vi "模拟器自动控制程序.vi"() -> ()   [LabVIEW 2012]
uses:
  <vilib>/Utility/error.llb/DialogType.ctl
  <vilib>/Platform/TimedLoop/XDataNode/timing_clust.ctl
  <vilib>/Platform/TimedLoop/XDataNode/nitl_modes.ctl
  <vilib>/Platform/TimedLoop/XDataNode/wakeup.ctl
  <vilib>/Instr/_visa.llb/VISA Configure Serial Port (Instr).vi
  <vilib>/DAQmx/create/channels.llb/DAQmx Create Channel (DO-Digital Output).vi
  <vilib>/Analysis/Matrix/Numeric/Conversions/Array To Matrix - RA2.vi
  <vilib>/Utility/file.llb/Write To Spreadsheet File (DBL).vi
  <vilib>/Platform/TimedLoop/XDataNode/XDataNode.xnode
  <vilib>/Platform/TimedLoop/XDataNode/XDNodeRunTimeDep.lvlib
  <vilib>/Analysis/Matrix/NI_Matrix.lvlib
  <vilib>/vision/NI_Vision_Development_Module.lvlib
  <vilib>/Analysis/NI_AALBase.lvlib
panel:
  out "Truster4":bool
  out "Truster 8":bool
  out "Truster  3":bool
  out "Truster 7":bool
  out "Truster 5":bool
  out "Truster  2":bool
  out "Truster 6":bool
  out "Truster1":bool
  out "alpha (deg)":dbl
  out "定位点信息":T1(array[cluster]) {"Aspect Ratio" format="%.2f"; "Orientation" format="%.2f"; "Area" format="%.2f"; "Object Center"."Y" format="%.2f"; "Object Center"."X" format="%.2f"}
  out "alpha":dbl
  out "计时参数":dbl
  in  "卫星模拟器":enum32{"初始化", "运行监测"}(tab)
  out "读取缓冲区":string
  out "电流校正模式":bool
  out "软件使能":bool caption="软件使能(启动/停止)"
  out "电流校正中":bool caption="电流校正完成"
  out "E2PROM初始化结果":bool
  out "E2初始化完成":bool
  out "串口通信错误":bool caption="串口通信故障"
  out "发送指令":string
  out "控制命令":string
  out "电机已启动":bool
  in  "采样率":i64=10
  in  "限制转速":dbl=500.0
  in  "ID号":u8=255 step=1 format="%#.0f"
  in  "最高转速":dbl=500.0
  in  "PWM周期":dbl=1599.0
  in  "最大力矩":dbl=2047.0
  in  "stop bits (10: 1 bit)":u16(ring)=10 caption="停止位" items=["1.0"=10, "1.5"=15, "2.0"=20]
  out "串口状态":bool
  in  "端口选择":refnum<visa-resource-name>="COM1"
  in  "波特率":u16(ring)=10 items=["   300", "   600", "   1200", "   2400", "   4800   ", "   9600", "   19200", "   38400", "   43000", "   56000", "   57600", "   115200"]
  in  "校验":enum16{"None", "Odd", "Even"}(ring)=enum."Even"
  in  "数据位":u16=8
  in  "打开":bool caption="stop"
  out "轨控信号":dbl
  in  "姿轨控开始":bool
  out "转速模式":bool
  out "转矩模式":bool
  out "故障":bool
  out "启停状态":bool
  in  "所需转角":dbl
  in  "存储波形":bool
  in  "显示波形 停止显示":bool
  in  "开始记录":bool
  out "动量轮转矩":dbl format="%#_6f"
  out "动量轮转速":dbl format="%#_4f"
  out "X速率(cm/s)":dbl
  out "Y速率(cm/s)":dbl
  out "Y偏移量 (cm)":dbl
  out "X偏移量 (cm)":dbl
  out "相对偏角(deg)":dbl
  out "角速度(deg/s)":dbl
  out "设备ID":u8=255
  in  "模式选择":u16(ring)=1 items=["电流校正模式", "转矩模式", "转速模式", "开环测试模式"]
  in  "模式选择":bool
  in  "写指令字":dbl
  in  "停止电机":bool
  in  "启动电机":bool
  out "波形图":cluster{"转矩反馈":dbl, "转速反馈":dbl}(graph)
  in  "所需X":dbl
  in  "退出程序":bool caption="停止电机 2"
  in  "Floating":bool
  in  "缩放比例 (像素/cm)":dbl=4.099468
  in  "X中心校正":dbl
  in  "Y中心校正":dbl
  in  "所需Y":dbl
  out "x >= y?":bool
  out "数值":dbl
  out "输出数组 6":dbl[](array[numeric])
  out "输出数组 7":dbl[](array[numeric])
  out "输出数组 10":dbl[](array[numeric])
  out "无符号字节数组 2":u8[](array[numeric])
  # "状态"
  # "设置"
  # "控制信号"
  # "参数确定"
  # "状态显示"
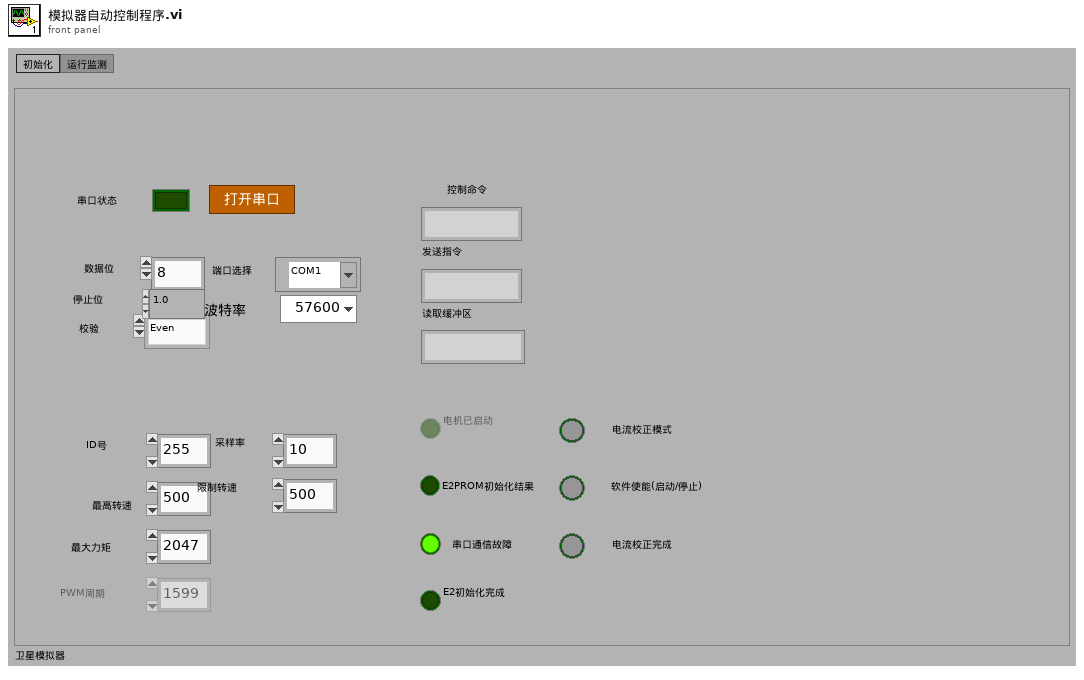
[diagram p1: front panel]
types:
  T1 = cluster{"Object Center":cluster{"X":sgl, "Y":sgl}, "Bounding Box":cluster{"X Left":i32, "Y Top":i32, "X Right":i32, "Y Bottom":i32}, "Area":sgl, "Orientation":sgl, "Aspect Ratio":sgl, "Nb Holes":i32}[]
  T2 = typedef "XDNodeRunTimeDep.lvlib/timing_clust.ctl" = cluster{"Expected End [f-1]":u64, "Actual End [f-1]":u64, "Finished Late? [f-1]":bool, "Expected End [i-1]":u64, "Actual End [i-1]":u64, "Finished Late? [i-1]":bool, "Expected Start [i]":u64, "Actual Start [i]":u64, "Expected Start [f]":u64, "Actual Start [f]":u64, "Source Name":string, "Structure Name":string, "Period":i64, "Deadline":i64, "Offset":i64, "Start":i64, "Priority":i32, "Timeout":i32, "Mode":T3, "Wakeup Reason":T4, "Error":errorcluster, "Source Type":string, "Secondary Source Type":string, "Global End Time":u64, "Global Start Time":u64, "Frame Duration":u64, "Iteration Duration":u64, "Assigned CPU":i32, "I/O Scan Engine Mode":u32}
  T3 = typedef "XDNodeRunTimeDep.lvlib/nitl_modes.ctl" = enum32{"No Change", "Process missed periods, maintain original phase", "Discard missed periods, maintain original phase", "Process missed periods, ignore original phase", "Discard missed periods, ignore original phase"}
  T4 = typedef "XDNodeRunTimeDep.lvlib/wakeup.ctl" = enum32{"Normal", "Aborted", "Asynchronous wakeup", "Timing source error", "Timed loop error", "Timeout"}
  T5 = cluster{"Objects":u16, "Threshold":i32, "Reject Border":bool, "Fill Holes":bool, "Min Object Size":bool, "Min Size":i32, "Max Object Size":bool, "Max Size":i32, "Show Search Area":bool, "Show Center":bool, "Show Bounding Box":bool}
  T6 = typedef "DialogType.ctl" = u16
  T7 = typedef "NI_Matrix.lvlib/RealMatrix.ctl" = dbl[][]
  T8 = typedef "IMAQ Image.ctl" = refnum<image>
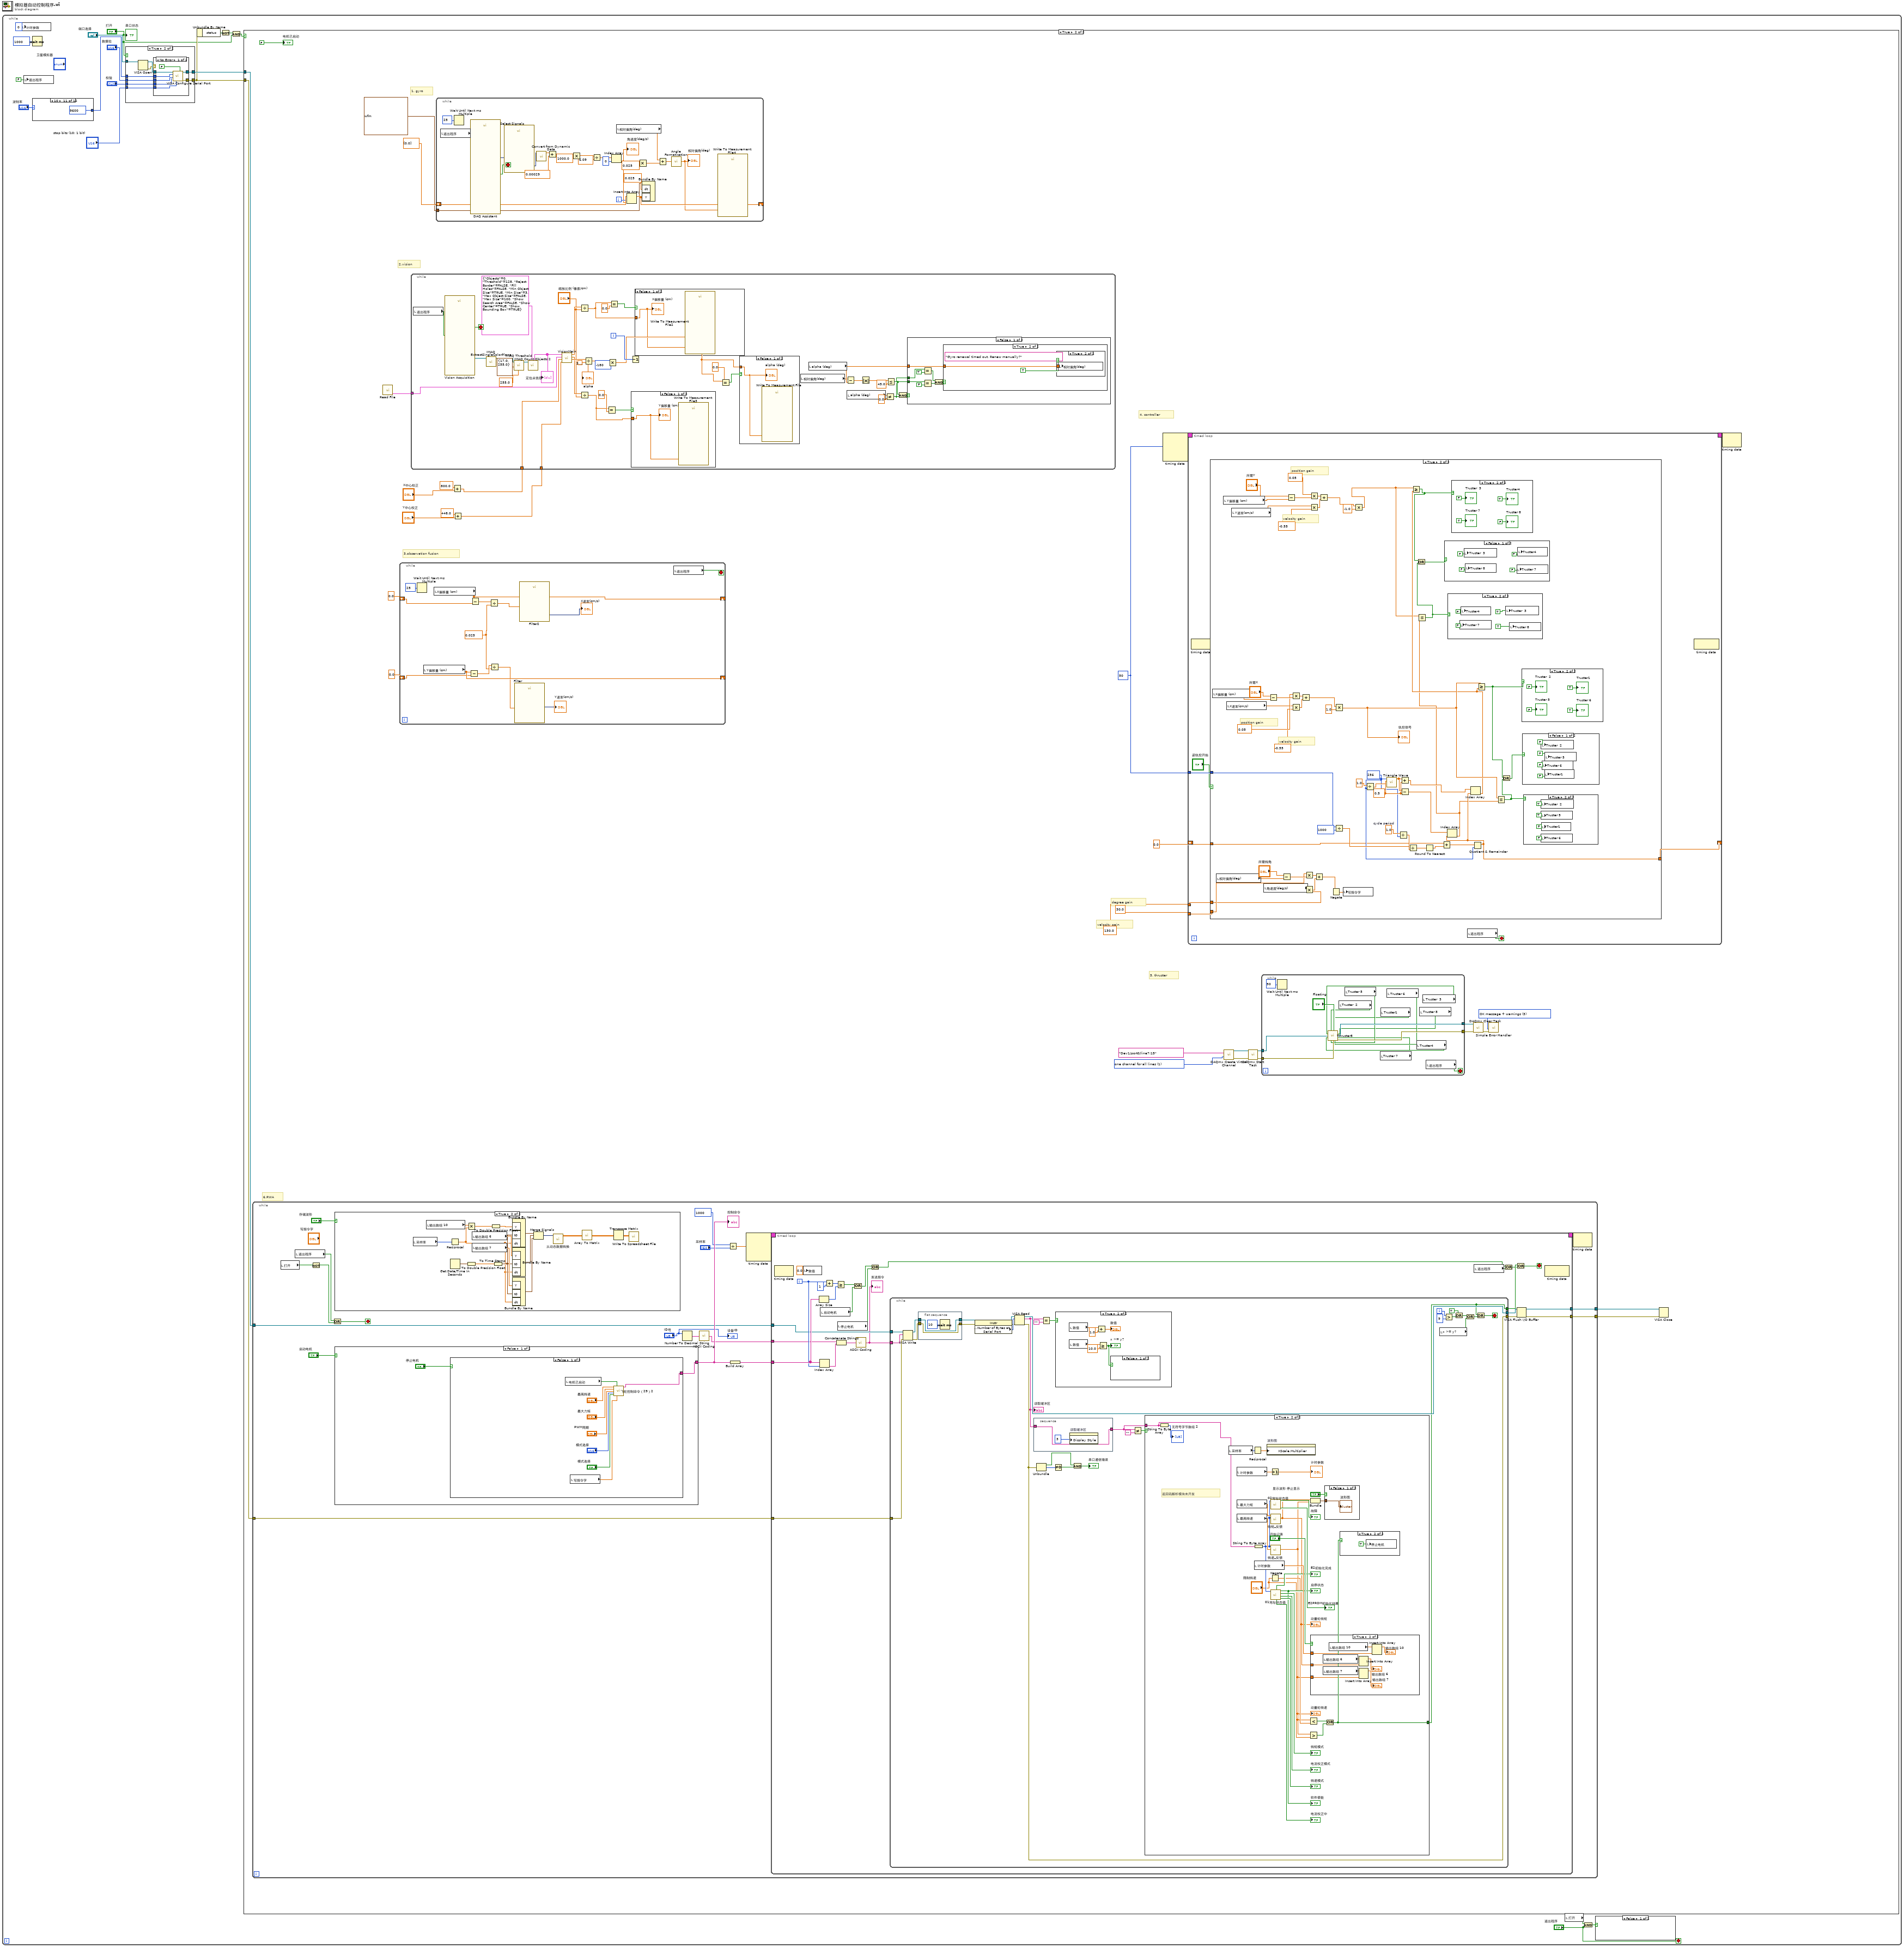
[diagram p0: block diagram]
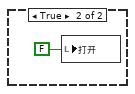
[diagram p2: hidden frame]
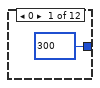
[diagram p5: hidden frame]
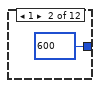
[diagram p6: hidden frame]
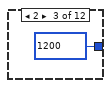
[diagram p7: hidden frame]
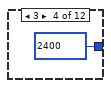
[diagram p8: hidden frame]
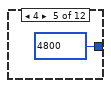
[diagram p9: hidden frame]
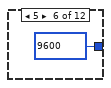
[diagram p10: hidden frame]
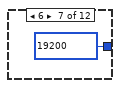
[diagram p11: hidden frame]
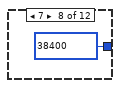
[diagram p12: hidden frame]
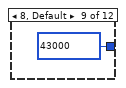
[diagram p13: hidden frame]
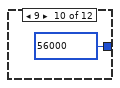
[diagram p14: hidden frame]
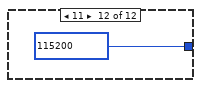
[diagram p15: hidden frame]
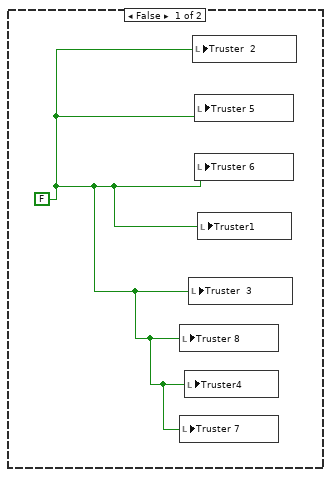
[diagram p17: hidden frame]
diagram:
  n1 = while {
    stop <- "退出程序" stop-if-true
    n2 = local write "计时参数"(0) -> ()
    n3 = local write "退出程序"(FALSE ("退出程序")) -> ()
    n4 = Wait (ms)(milliseconds to wait=u32 1000 ("等待时间（毫秒）")) -> ()  [unwired: 1 out]
    n5 = case shown="10" "波特率" {
      tunnel: [300 600 1200 2400 4800 9600 19200 38400 43000 56000 9600 115200] -> w17
      frame 0 {
      }
      frame 1 {
      }
      frame 2 {
      }
      frame 3 {
      }
      frame 4 {
      }
      frame 5 {
      }
      frame 6 {
      }
      frame 7 {
      }
      frame 8, Default {
      }
      frame 9 {
      }
      frame 10 {
      }
      frame 11 {
      }
    }
    n6 = case shown="True" "打开" {
      tunnel: w17 -> [_ w28]
      tunnel: "数据位" -> [_ w27]
      tunnel: "校验" -> [_ w26]
      tunnel: "端口选择" -> [_ w25]
      tunnel: [_ w22] -> w7
      tunnel: [_ w21] -> w6
      tunnel: "stop bits (10: 1 bit)" -> [_ w20]
      frame False {
      }
      frame True {
        n7 = VISA Open(VISA resource name=w25) -> (VISA resource name=w24:refnum<visa-resource-name>, error out=w23:errorcluster)  [unwired: 1 in, 3 out]
        n8 = case shown="No Error" w23 {
          tunnel: w28 -> [w36 _]
          tunnel: w27 -> [w35 _]
          tunnel: w26 -> [w34 _]
          tunnel: w24 -> [w33 _]
          tunnel: [w32 _] -> w22
          tunnel: [w31 _] -> w21
          tunnel: w20 -> [w30 _]
          frame No Error {
            n9 = call-poly "VISA Configure Serial Port"("VISA resource name"=w33, "Enable Termination\nChar (T)"=FALSE ("Enable Termination\nChar (T)"), "baud rate (9600)"=w36, "data bits (8)"=w35, "parity (0:none)"=w34, "stop bits (10: 1 bit)"=w30) -> ("VISA resource name out"=w32:refnum<visa-resource-name>, "error out"=w31:errorcluster)  [unwired: 2 in, 6 out]
          }
          frame Error {
          }
        }
      }
    }
    n10 = Unbundle By Name(w6) -> ("status"=w12:bool)
    n11 = Not(x=w12) -> (.not. x?=w11:bool)
    n12 = And(x=w11, y="打开") -> (x .and. y?=w8:bool)
    n13 = case shown="True" w8 {
      tunnel: w7 -> [_ w77]
      tunnel: w6 -> [_ w76]
      frame False {
      }
      frame True {
        w55 = 1 items=["one channel for each line", "one channel for all lines"] ("line grouping")
        w57 = T6 3 items=["no dialog", "OK message", "continue or stop message", "OK message + warnings", "continue/stop + warnings"] ("type of dialog (OK msg:1)")
        w51 = 50
        # "5. thruster"
        # "6.RWA"
        # "4. controller"
        # "3.observation fusion"
        # "2.vision"
        # "1. gyro"
        # "velocity gain"
        # "degree gain"
        n14 = while {
          tunnel: [w292] -> w79
          tunnel: [w291] -> w78
          tunnel: w77 -> [w290]
          tunnel: w76 -> [w289]
          stop <- w285 stop-if-true
          n15 = local read "打开"() -> (w288:bool)
          n16 = local read "退出程序"() -> (w287:bool)
          n17 = Not(x=w288) -> (.not. x?=w286:bool)
          n18 = Or(x=w287, y=w286) -> (x .or. y?=w285:bool)
          n19 = case shown="True" "存储波形" {
            frame False {
            }
            frame True {
              n20 = local read "采样率"() -> (w314:i64)
              n21 = local read "输出数组 10"() -> (w307:dbl[])
              n22 = Reciprocal(x=w314) -> (1/x=w309:dbl)
              n23 = Get Date/Time In Seconds() -> (seconds since 1Jan1904=w318:timestamp)
              n24 = Multiply(x=w307, y=w309) -> (x*y=w308:dbl[])
              n25 = To Double Precision Float(number=w318) -> (double precision float=w317:dbl)
              n26 = local read "输出数组 6"() -> (w316:dbl[])
              n27 = local read "输出数组 7"() -> (w315:dbl[])
              n28 = To Double Precision Float(number=w308) -> (double precision float=w306:dbl[])
              n29 = To Time Stamp(1:w317) -> (0:w310:timestamp)
              n30 = Bundle By Name("Y"=w306, "t0"=w310, "dt"=w309) -> (w311:waveform(dbl))  [unwired: 1 out]
              n31 = Bundle By Name("Y"=w316, "t0"=w310, "dt"=w309) -> (w312:waveform(dbl))  [unwired: 1 out]
              n32 = Bundle By Name("Y"=w315, "t0"=w310, "dt"=w309) -> (w313:waveform(dbl))  [unwired: 1 out]
              n33 = Merge Signals(w311, w312, w313) -> (w305:dynamicdata)
              n34 = call "从动态数据转换"("Dynamic Data Type"=w305) -> ("Array"=w304:dbl[][])  [unwired: 3 in]
              n35 = call-poly <vilib>:"Array To Matrix.vi"("Real 2D Array"=w304) -> ("Real Matrix"=w303:T7)
              n36 = Transpose Matrix(1:w303) -> (0:w302:T7)
              n37 = call-poly <vilib>:"Write To Spreadsheet File.vi"("2D data"=w302) -> ()  [unwired: 7 in, 1 out]
            }
          }
          n38 = case shown="False" "启动电机" {
            tunnel: [w434 w449] -> w300
            frame False {
              n39 = case shown="False" "停止电机" {
                tunnel: [w442 "v0"] -> w434
                frame False {
                  n40 = local read "电机已启动"() -> (w436:bool)
                  n41 = local read "写指令字"() -> (w435:dbl)
                  n42 = call "飞轮控制命令（29）2.vi"("最高转速"="最高转速", "电机启动控制指令"=w436, "力矩最大值(uNm)"="最大力矩", "pwmperiod"="PWM周期", "模式选择"="模式选择", "模式确定"="模式选择", "写指令字"=w435) -> ("字符串"=w442:string)  [unwired: 8 in]
                }
                frame True {
                  n43 = local write "电机已启动"(FALSE) -> ()
                  n44 = local write "启动电机"(FALSE ("停止电机")) -> ()
                  n45 = local write "停止电机"(FALSE ("停止电机")) -> ()
                }
              }
            }
            frame True {
              n46 = local write "电机已启动"(TRUE) -> ()
              n47 = local write "启动电机"(FALSE) -> ()
              n48 = call <vilib>:"Space Constant.vi"() -> ("String"=w453:string)
              n49 = Concatenate Strings(w453, "05" ("字符串"), w453, "22" ("字符串"), w453, "01" ("字符串")) -> (w449:string)
            }
          }
          "控制命令" <- w300
          n50 = Number To Decimal String(number="ID号") -> (decimal integer string=w284:string)  [unwired: 1 in]
          n51 = call "ASCII Coding.vi"("cmd"=w284) -> ("cmd sent"=w282:string)
          n52 = Divide(x=i64 1000 ("Period"), y="采样率") -> (x/y=w296:dbl)
          n53 = Build Array(w300) -> (w297:string[])
          n54 = node-c288(w296) -> (w299:T2)  [unwired: 3 in]
          n55 = timed-loop {
            timing: w299 -> [_]
            timing-out: [_] -> w298
            tunnel: w297 -> [w340]
            tunnel: w282 -> [w336]
            tunnel: [w333] -> w292
            tunnel: [w332] -> w291
            tunnel: w290 -> [w331]
            tunnel: w289 -> [w330]
            i -> [w339]
            stop <- w321 stop-if-true
            n56 = node-c288() -> ()  [unwired: 1 in, 1 out]
            n57 = local write "数值"(0.0 ("y")) -> ()
            n58 = Array Size(array=w340) -> (size(s)=w342:i32)
            n59 = Index Array(array=w340, index=w339) -> (element=w341:string)
            n60 = local read "启动电机"() -> (w328:bool)
            n61 = Add(x=w339, y=1) -> (x+y=w343:i32)
            n62 = Greater Or Equal?(x=w343, y=w342) -> (x >= y?=w329:bool)
            n63 = Concatenate Strings(w336, w341) -> (w320:string)
            n64 = local read "停止电机"() -> (w327:bool)
            n65 = Or(x=w329, y=w328) -> (x .or. y?=w326:bool)
            n66 = call "ASCII Coding.vi"("cmd"=w320) -> ("cmd sent"=w319:string)
            "发送指令" <- w319
            n67 = Or(x=w326, y=w327) -> (x .or. y?=w324:bool)
            n68 = while {
              tunnel: [w371] -> w334
              tunnel: [w361] -> w335
              tunnel: w319 -> [w365]
              tunnel: w331 -> [w347]
              tunnel: w330 -> [w346]
              tunnel: [w345] -> w323
              i -> [w370]
              stop <- w354 stop-if-true
              n69 = VISA Write(VISA resource name=w347, write buffer=w365, error in (no error)=w346) -> (VISA resource name out=w352:refnum<visa-resource-name>, error out=w349:errorcluster)  [unwired: 1 out]
              n70 = flat-sequence {
                tunnel: w352 -> [w377]
                tunnel: [w377] -> w351
                tunnel: [w376] -> w350
                tunnel: w349 -> [w376]
                frame #0 {
                  n71 = Wait (ms)(milliseconds to wait=i64 10 ("Period")) -> ()  [unwired: 1 out]
                }
              }
              n72 = property class="Instr"(reference=w351, error in=w350) -> (reference out=w373:refnum<visa-resource-name>, error out=w372:errorcluster, "Serial Settings:Number of Bytes at Serial Port"=w374:u32)
              n73 = VISA Read(VISA resource name=w373, byte count=w374, error in (no error)=w372) -> (VISA resource name out=w371:refnum<visa-resource-name>, read buffer=w364:string, error out=w361:errorcluster)  [unwired: 1 out]
              "读取缓冲区" <- w364
              n74 = stacked-sequence {
                tunnel: [w418] -> w363
                tunnel: w364 -> [w418]
                frame #0 {
                  n75 = property on="读取缓冲区" class="Str"("Display Style"=u32 3 ("显示样式")) -> ()  [unwired: 2 in, 2 out]
                }
              }
              n76 = Unbundle(w361) -> ("status"=w358:bool, "code"=w360:i32)  [unwired: 1 out]
              n77 = Equal?(x=w364, y="") -> (x = y?=w367:bool)
              n78 = Not Equal To 0?(x=w360) -> (x != 0?=w359:bool)
              n79 = case shown="True" w367 {
                frame False {
                  n80 = local write "数值"(0.0 ("数值")) -> ()
                }
                frame True {
                  n81 = local read "数值"() -> (w420:dbl)
                  n82 = local read "数值"() -> (w425:dbl)
                  n83 = Add(x=w420, y=1.0) -> (x+y=→"数值":dbl)
                  n84 = Greater Or Equal?(x=w425, y=10.0) -> (x >= y?=w423:bool)
                  "x >= y?" <- w423
                  n85 = case shown="False" w423 {
                    frame False {
                    }
                    frame True {
                      n86 = local write "打开"(FALSE) -> ()
                    }
                  }
                }
              }
              n87 = And(x=w358, y=w359) -> (x .and. y?=→"串口通信错误":bool)
              n88 = Not Equal?(x=w363, y="") -> (x != y?=w353:bool)
              n89 = case shown="True" w353 {
                tunnel: w363 -> [_ w405]
                tunnel: [_ w404] -> w345
                frame False {
                }
                frame True {
                  # "返回码解析模块未开发"
                  n90 = String To Byte Array(string=w405) -> (unsigned byte array=→"无符号字节数组 2":u8[])
                  n91 = local read "采样率"() -> (w401:i64)
                  n92 = local read "计时参数"() -> (w398:dbl)
                  n93 = local read "最大力矩"() -> (w386:dbl)
                  n94 = local read "最高转速"() -> (w384:dbl)
                  n95 = Reciprocal(x=w401) -> (1/x=w400:dbl)
                  n96 = String To Byte Array(string=w405) -> (unsigned byte array=w383:u8[])
                  n97 = local read "计时参数"() -> (w395:dbl)
                  n98 = property on="波形图" class="WFChart (strict)"("XScale.Multiplier"=w400) -> ()  [unwired: 2 in, 2 out]
                  n99 = Increment(x=w398) -> (x+1=→"计时参数":dbl)
                  n100 = Negate(x="限制转速") -> (-x=w382:dbl)
                  n101 = call "02地址状态值.vi"("unsigned byte array"=w383) -> ("E2初始化失败"=→"E2PROM初始化结果":bool, "故障"=→"故障":bool)  [unwired: 9 in]
                  n102 = call "转矩_反馈.vi"("unsigned byte array"=w383, "最大转矩"=w386) -> ("转矩反馈"=w385:dbl)  [unwired: 9 in]
                  "动量轮转矩" <- w385
                  n103 = call "转速_反馈.vi"("最高转速"=w384, "unsigned byte array"=w383) -> ("转速反馈"=w381:dbl)  [unwired: 9 in]
                  "动量轮转速" <- w381
                  n104 = call "01地址状态值.vi"("unsigned byte array"=w383) -> ("E2初始化完成"=→"E2初始化完成":bool, "电流校正完成"=→"电流校正中":bool, "启停状态"=→"软件使能" →"启停状态":bool, "转矩模式"=→"转矩模式":bool, "电流校正"=→"电流校正模式":bool, "转速模式"=→"转速模式":bool)  [unwired: 4 in]
                  n105 = Less?(x=w381, y=w382) -> (x < y?=w378:bool)
                  n106 = Greater?(x=w381, y="限制转速") -> (0:w379:bool)
                  n107 = Bundle("转矩反馈"=w385, "转速反馈"=w381) -> (w402:cluster{"转矩反馈":dbl, "转速反馈":dbl})  [unwired: 1 out]
                  n108 = case shown="True" "开始记录" {
                    tunnel: w385 -> [_ w409]
                    tunnel: w381 -> [_ w408]
                    tunnel: w395 -> [_ w407]
                    frame False {
                    }
                    frame True {
                      n109 = local read "输出数组 6"() -> (w414:dbl[])
                      n110 = local read "输出数组 7"() -> (w412:dbl[])
                      n111 = local read "输出数组 10"() -> (w410:dbl[])
                      n112 = Insert Into Array(array=w414, new element=w409) -> (→"输出数组 6":dbl[])  [unwired: 1 in]
                      n113 = Insert Into Array(array=w412, new element=w408) -> (→"输出数组 7":dbl[])  [unwired: 1 in]
                      n114 = Insert Into Array(array=w410, new element=w407) -> (→"输出数组 10":dbl[])  [unwired: 1 in]
                    }
                  }
                  n115 = case shown="False" "显示波形 停止显示" {
                    tunnel: w402 -> [w416 _]
                    frame False {
                      "波形图" <- w416
                    }
                    frame True {
                    }
                  }
                  n116 = Or(x=w378, y=w379) -> (x .or. y?=w404:bool)
                  n117 = case shown="True" w404 {
                    frame False {
                    }
                    frame True {
                      n118 = local write "停止电机"(TRUE ("停止电机")) -> ()
                    }
                  }
                }
              }
              n119 = local read "x >= y?"() -> (w356:bool)
              n120 = Greater?(x=w370, y=9) -> (0:w348:bool)
              n121 = Or(x=TRUE, y=w348) -> (x .or. y?=w366:bool)
              n122 = Or(x=w366, y=w356) -> (x .or. y?=w355:bool)
              n123 = Or(x=w345, y=w355) -> (x .or. y?=w354:bool)
            }
            n124 = local read "退出程序"() -> (w325:bool)
            n125 = Or(x=w324, y=w325) -> (x .or. y?=w322:bool)
            n126 = Or(x=w323, y=w322) -> (x .or. y?=w321:bool)
            n127 = VISA Flush I/O Buffer(VISA resource name=w334, error in (no error)=w335) -> (VISA resource name out=w333:refnum<visa-resource-name>, error out=w332:errorcluster)  [unwired: 1 out]
            n128 = node-c288() -> ()  [unwired: 1 in, 1 out]
          }
          n129 = node-c288(w298) -> ()  [unwired: 1 out]
          "设备ID" <- "ID号"
        }
        n130 = call "Read File.vi"() -> ("Objects"=w74:T1)  [unwired: 1 in, 1 out]
        n131 = while {
          shift-right: [w275] -> _
          shift-left: 0.0 ("X偏移量 (cm)") -> [w274]
          shift-right: [w272] -> _
          shift-left: 0.0 ("Y偏移量 (cm)") -> [w271]
          stop <- w280 stop-if-true
          w273 = 0.025 ("y")
          n132 = Wait Until Next ms Multiple(millisecond multiple=u32 25) -> ()  [unwired: 1 out]
          n133 = local read "Y偏移量 (cm)"() -> (w272:dbl)
          n134 = local read "X偏移量 (cm)"() -> (w275:dbl)
          n135 = Subtract(x=w272, y=w271) -> (x-y=w277:dbl)
          n136 = Subtract(x=w275, y=w274) -> (x-y=w278:dbl)
          n137 = Divide(x=w278, y=w273) -> (x/y=w269:dbl)
          n138 = Divide(x=w277, y=w273) -> (x/y=w270:dbl)
          n139 = call "Filter"("Signal"=w270) -> ("Filtered Signal"=→"Y速率(cm/s)":dynamicdata)  [unwired: 9 in, 1 out]
          n140 = call "Filter2"("Signal"=w269) -> ("Filtered Signal"=→"X速率(cm/s)":dynamicdata)  [unwired: 9 in, 1 out]
          n141 = local read "退出程序"() -> (w280:bool)
        }
        n142 = while {
          shift-right: [w253] -> _
          shift-left: dbl[] [0.0] -> [w254]
          tunnel: waveform(dbl) {"t0"=timestamp(0 s since 1904-01-01), "dt"=1.0, "Y"=[]} ("waveform") -> [w251]
          i -> [w252]
          stop <- w268 stop-if-true
          n143 = local read "退出程序"() -> (w248:bool)
          n144 = Wait Until Next ms Multiple(millisecond multiple=u32 25 ("y")) -> ()  [unwired: 1 out]
          n145 = call "DAQ Assistant"("stop (F)"=w248) -> ("data"=w246:dynamicdata, "stopped"=w268:bool)  [unwired: 15 in, 2 out]
          n146 = call "Select Signals"("Signals"=w246) -> ("Signal Out"=w247:dynamicdata)  [unwired: 9 in, 1 out]
          n147 = call "Convert from Dynamic Data"("Dynamic Data Type"=w247) -> ("Array"=w259:dbl[])  [unwired: 3 in]
          n148 = Add(x=w259, y=0.00029) -> (x+y=w257:dbl[])
          n149 = Multiply(x=w257, y=1000.0) -> (x*y=w267:dbl[])
          n150 = Divide(x=w267, y=6.09) -> (x/y=w261:dbl[])
          n151 = Index Array(array=w261, index=0) -> (element=w249:dbl)
          "角速度(deg/s)" <- w249
          n152 = local read "相对偏角(deg)"() -> (w256:dbl)
          n153 = Insert Into Array(array=w254, index=w252, new element=w249) -> (w253:dbl[])
          n154 = Multiply(x=w249, y=0.025) -> (x*y=w262:dbl)
          n155 = Bundle By Name(cluster=w251, "dt"=0.025, "Y"=w253) -> ()  [unwired: 1 out]
          n156 = Add(x=w256, y=w262) -> (x+y=w250:dbl)
          n157 = call "Angle Formatization.vi"("Alpha"=w250) -> ("Alpha Formatized"=w245:dbl)
          "相对偏角(deg)" <- w245
          n158 = call "Write To Measurement File4"("Signals"=w245) -> ()  [unwired: 16 in, 3 out]
        }
        n159 = Add(x=800.0 ("c_x"), y="X中心校正") -> (x+y=w69:dbl)
        n160 = Add(x=448.0 ("c_y"), y="Y中心校正") -> (x+y=w66:dbl)
        n161 = while {
          tunnel: w74 -> [w204]
          tunnel: w66 -> [w198]
          tunnel: w69 -> [w197]
          i -> [w200]
          stop <- w214 stop-if-true
          n162 = local read "退出程序"() -> (w206:bool)
          n163 = call "Vision Acquisition"("Stop (F)"=w206) -> ("Image Out"=w210:T8, "Stopped"=w214:bool)  [unwired: 24 in, 1 out]
          n164 = call "IMAQ ExtractSingleColorPlane"("Image Src"=w210) -> ("Image Dst Out"=w195:T8)  [unwired: 9 in, 1 out]
          n165 = call "IMAQ Threshold"("Replace Value"=sgl 255.0 ("replace value"), "Range"=cluster{"lower value":sgl, "upper value":sgl} {"lower value"=17.0, "upper value"=255.0} ("threshold"), "Image Src"=w195) -> ("Image Dst Out"=w211:T8)  [unwired: 7 in, 1 out]
          n166 = call "IMAQ Count Objects 2"("Settings"=T5 {"Objects"=0, "Threshold"=128, "Reject Border"=FALSE, "Fill Holes"=FALSE, "Min Object Size"=TRUE, "Min Size"=3, "Max Object Size"=FALSE, "Max Size"=100, "Show Search Area"=FALSE, "Show Center"=TRUE, "Show Bounding Box"=TRUE}, "Image"=w211) -> ("Objects"=w205:T1)  [unwired: 5 in, 4 out]
          "定位点信息" <- w205
          n167 = call "VisionMain.vi"("Y Center"=w198, "X Center"=w197, "Original Plots"=w204, "Plots Captured"=w205) -> ("alpha"=w203:dbl, "dy"=w202:dbl, "dx"=w201:dbl)  [unwired: 5 in]
          "alpha" <- w203
          n168 = Divide(x=w201, y="缩放比例 (像素/cm)") -> (x/y=w189:dbl)
          n169 = Divide(x=w202, y="缩放比例 (像素/cm)") -> (x/y=w186:dbl)
          n170 = Divide(x=w203, y=3.141592653589793) -> (x/y=w208:dbl)
          n171 = Equal?(x=w186, y=0.0) -> (x = y?=w187:bool)
          n172 = Multiply(x=w208, y=-180) -> (x*y=w192:dbl)
          n173 = Equal?(x=w189, y=0.0) -> (x = y?=w190:bool)
          n174 = Decrement(x=w200) -> ()  [unwired: 1 out]
          n175 = case shown="False" w187 {
            tunnel: w186 -> [w227 _]
            frame False {
              n176 = call "Write To Measurement File3"("Signals"=w227) -> ()  [unwired: 16 in, 3 out]
              "Y偏移量 (cm)" <- w227
            }
            frame True {
            }
          }
          n177 = case shown="False" w190 {
            tunnel: w189 -> [w228 _]
            frame False {
              n178 = call "Write To Measurement File2"("Signals"=w228) -> ()  [unwired: 16 in, 3 out]
              "X偏移量 (cm)" <- w228
            }
            frame True {
            }
          }
          n179 = Equal?(x=w192, y=0.0) -> (x = y?=w193:bool)
          n180 = case shown="False" w193 {
            tunnel: w192 -> [w229 _]
            frame False {
              n181 = call "Write To Measurement File"("Signals"=w229) -> ()  [unwired: 16 in, 3 out]
              "alpha (deg)" <- w229
            }
            frame True {
            }
          }
          n182 = local read "相对偏角(deg)"() -> (w176:dbl)
          n183 = local read "alpha (deg)"() -> (w180:dbl)
          n184 = Subtract(x=w176, y=w180) -> (x-y=w177:dbl)
          n185 = local read "alpha (deg)"() -> (w182:dbl)
          n186 = Absolute Value(x=w177) -> (abs(x)=w178:dbl)
          n187 = Not Equal?(x=w182, y=0.0) -> (x != y?=w184:bool)
          n188 = Less Or Equal?(x=w178, y=45.0) -> (x <= y?=w185:bool)
          n189 = And(x=w185, y=w184) -> (x .and. y?=w181:bool)
          n190 = case shown="False" w181 {
            tunnel: w180 -> [w215 w226]
            tunnel: w184 -> [w217 _]
            tunnel: w185 -> [w216 _]
            frame False {
              n191 = Equal?(x=w217, y=TRUE) -> (x = y?=w221:bool)
              n192 = Equal?(x=w216, y=FALSE) -> (x = y?=w220:bool)
              n193 = And(x=w221, y=w220) -> (x .and. y?=w218:bool)
              n194 = case shown="True" w218 {
                tunnel: w215 -> [_ w224]
                frame False {
                }
                frame True {
                  (unwired) "Gyro renewal timed out. Renew manually?" ("message")
                  n195 = case shown="True" TRUE {
                    tunnel: w224 -> [_ w225]
                    frame False {
                    }
                    frame True {
                      n196 = local write "相对偏角(deg)"(w225) -> ()
                    }
                  }
                }
              }
            }
            frame True {
              n197 = local write "相对偏角(deg)"(w226) -> ()
            }
          }
        }
        n198 = node-c288(w51) -> (w53:T2)  [unwired: 3 in]
        n199 = timed-loop {
          tunnel: 30.0 ("degree gain") -> [w87]
          tunnel: 130.0 ("angular velocity gain") -> [w86]
          shift-right: [w85] -> _
          shift-left: 0.0 -> [w84]
          tunnel: w51 -> [w83]
          timing: w53 -> [_]
          timing-out: [_] -> w52
          stop <- w82 stop-if-true
          n200 = node-c288() -> ()  [unwired: 1 in, 1 out]
          n201 = case shown="True" "姿轨控开始" {
            tunnel: w87 -> [_ w143]
            tunnel: w86 -> [_ w142]
            tunnel: [_ w110] -> w85
            tunnel: w84 -> [_ w109]
            tunnel: w83 -> [_ w108]
            frame False {
              w88 = FALSE ("Truster 6")
              n202 = local write "Truster 8"(w88) -> ()
              n203 = local write "Truster 7"(w88) -> ()
              n204 = local write "Truster4"(w88) -> ()
              n205 = local write "Truster  3"(w88) -> ()
              n206 = local write "Truster  2"(w88) -> ()
              n207 = local write "Truster 5"(w88) -> ()
              n208 = local write "Truster 6"(w88) -> ()
              n209 = local write "Truster1"(w88) -> ()
            }
            frame True {
              w114 = 256 ("samples")
              w122 = 1.0  # cycle period
              w126 = 0.5 ("amplitude")
              # "position gain"
              # "velocity gain"
              # "velocity gain"
              # "position gain"
              n210 = local read "X偏移量 (cm)"() -> (w133:dbl)
              n211 = local read "相对偏角(deg)"() -> (w137:dbl)
              n212 = local read "Y偏移量 (cm)"() -> (w99:dbl)
              n213 = local read "X速率(cm/s)"() -> (w131:dbl)
              n214 = local read "Y速率(cm/s)"() -> (w97:dbl)
              n215 = local read "角速度(deg/s)"() -> (w136:dbl)
              n216 = Subtract(x="所需X", y=w133) -> (x-y=w135:dbl)
              n217 = Subtract(x="所需转角", y=w137) -> (x-y=w145:dbl)
              n218 = Subtract(x="所需Y", y=w99) -> (x-y=w104:dbl)
              n219 = Multiply(x=0.05 ("degree gain"), y=w135) -> (x*y=w128:dbl)
              n220 = Multiply(x=w131, y=-0.55) -> (x*y=w129:dbl)
              n221 = Add(x=w128, y=w129) -> (x+y=w106:dbl)
              n222 = Multiply(x=w143, y=w145) -> (x*y=w144:dbl)
              n223 = Multiply(x=w136, y=w142) -> (x*y=w141:dbl)
              n224 = Multiply(x=0.05 ("degree gain"), y=w104) -> (x*y=w101:dbl)
              n225 = Multiply(x=w97, y=-0.55) -> (x*y=w102:dbl)
              n226 = Add(x=w144, y=w141) -> (x+y=w139:dbl)
              n227 = Add(x=w101, y=w102) -> (x+y=w89:dbl)
              n228 = Negate(x=w139) -> (-x=w138:dbl)
              n229 = Multiply(x=w106, y=1.0) -> (x*y=w105:dbl)
              "轨控信号" <- w105
              n230 = Divide(x=w108, y=u32 1000) -> (x/y=w120:dbl)
              n231 = local write "写指令字"(w138) -> ()
              n232 = Multiply(x=w89, y=-1.0) -> (x*y=w90:dbl)
              n233 = Divide(x=1.0 ("amplitude"), y=w114) -> (x/y=w123:dbl)
              n234 = call <vilib>:"Triangle Wave.vi"("samples"=w114, "amplitude"=w126, "frequency"=w123) -> ("triangle wave"=w127:dbl[])  [unwired: 2 in, 2 out]
              n235 = Divide(x=w122, y=w114) -> (x/y=w121:dbl)
              n236 = Add(x=w127, y=w126) -> (x+y=w118:dbl[])
              n237 = Subtract(x=w127, y=w126) -> (x-y=w117:dbl[])
              n238 = Divide(x=w120, y=w121) -> (x/y=w119:dbl)
              n239 = Round To Nearest(number=w119) -> (nearest integer value=w116:dbl)
              n240 = Add(x=w109, y=w116) -> (x+y=w115:dbl)
              n241 = Quotient & Remainder(x=w115, y=w114) -> (x-y*floor(x/y)=w110:dbl)  [unwired: 1 out]
              n242 = Index Array(array=w117, index=w110) -> (element=w95:dbl)
              n243 = Less Or Equal?(x=w90, y=w95) -> (x <= y?=w93:bool)
              n244 = case shown="True" w93 {
                frame False {
                }
                frame True {
                  n245 = local write "Truster 7"(FALSE ("Truster 6")) -> ()
                  n246 = local write "Truster4"(FALSE ("Truster 6")) -> ()
                  n247 = local write "Truster  3"(TRUE ("Truster 6")) -> ()
                  n248 = local write "Truster 8"(TRUE ("Truster 6")) -> ()
                }
              }
              n249 = Index Array(array=w118, index=w110) -> (element=w96:dbl)
              n250 = Greater Or Equal?(x=w90, y=w96) -> (x >= y?=w94:bool)
              n251 = Or(x=w94, y=w93) -> (x .or. y?=w92:bool)
              n252 = case shown="False" w92 {
                frame False {
                  n253 = local write "Truster  3"(FALSE ("Truster 6")) -> ()
                  n254 = local write "Truster 8"(FALSE ("Truster 6")) -> ()
                  n255 = local write "Truster 7"(FALSE ("Truster 6")) -> ()
                  n256 = local write "Truster4"(FALSE ("Truster 6")) -> ()
                }
                frame True {
                }
              }
              n257 = case shown="True" w94 {
                frame False {
                }
                frame True {
                  "Truster4" <- TRUE ("Truster 6")
                  "Truster 8" <- FALSE ("Truster 6")
                  "Truster  3" <- FALSE ("Truster 6")
                  "Truster 7" <- TRUE ("Truster 6")
                }
              }
              n258 = Greater Or Equal?(x=w105, y=w96) -> (x >= y?=w113:bool)
              n259 = Less Or Equal?(x=w105, y=w95) -> (x <= y?=w112:bool)
              n260 = Or(x=w113, y=w112) -> (x .or. y?=w111:bool)
              n261 = case shown="True" w113 {
                frame False {
                }
                frame True {
                  "Truster1" <- TRUE ("Truster 6")
                  "Truster 6" <- TRUE ("Truster 6")
                  "Truster  2" <- FALSE ("Truster 6")
                  "Truster 5" <- FALSE ("Truster 6")
                }
              }
              n262 = case shown="False" w111 {
                frame False {
                  n263 = local write "Truster  2"(FALSE ("Truster 6")) -> ()
                  n264 = local write "Truster 6"(FALSE ("Truster 6")) -> ()
                  n265 = local write "Truster1"(FALSE ("Truster 6")) -> ()
                  n266 = local write "Truster 5"(FALSE ("Truster 6")) -> ()
                }
                frame True {
                }
              }
              n267 = case shown="True" w112 {
                frame False {
                }
                frame True {
                  n268 = local write "Truster  2"(TRUE ("Truster 6")) -> ()
                  n269 = local write "Truster 5"(TRUE ("Truster 6")) -> ()
                  n270 = local write "Truster 6"(FALSE ("Truster 6")) -> ()
                  n271 = local write "Truster1"(FALSE ("Truster 6")) -> ()
                }
              }
            }
          }
          n272 = local read "退出程序"() -> (w82:bool)
          n273 = node-c288() -> ()  [unwired: 1 in, 1 out]
        }
        n274 = call-poly <vilib>:"DAQmx Create Virtual Channel.vi"("lines"=tag "Dev1/port0/line7:15" ("Lines"), "line grouping"=w55) -> ("task out"=w60:refnum<k21>, "error out"=w59:errorcluster)  [unwired: 12 in]
        n275 = call <vilib>:"DAQmx Start Task.vi"("task/channels in"=w60, "error in"=w59) -> ("task out"=w62:refnum<k21>, "error out"=w65:errorcluster)  [unwired: 12 in]
        n276 = while {
          tunnel: w65 -> [w240]
          tunnel: [w241] -> w64
          tunnel: w62 -> [w243]
          tunnel: [w242] -> w61
          stop <- w244 stop-if-true
          n277 = Wait Until Next ms Multiple(millisecond multiple=u32 50) -> ()  [unwired: 1 out]
          n278 = local read "Truster  2"() -> (w237:bool)
          n279 = local read "Truster 5"() -> (w238:bool)
          n280 = local read "Truster 7"() -> (w230:bool)
          n281 = local read "Truster1"() -> (w236:bool)
          n282 = local read "Truster 6"() -> (w235:bool)
          n283 = local read "Truster4"() -> (w231:bool)
          n284 = local read "Truster 8"() -> (w232:bool)
          n285 = local read "Truster  3"() -> (w233:bool)
          n286 = call "Thruster8.vi"("Thruster 2"=w237, "Truster1"=w236, "Floating"="Floating", "Thruster 3"=w233, "Thruster 8"=w232, "task in"=w243, "Thruster 4"=w231, "Thruster 7"=w230, "Thruster 5"=w238, "error in"=w240, "Thruster 6"=w235) -> ("task out"=w242:refnum<k21>, "error out"=w241:errorcluster)  [unwired: 3 in]
          n287 = local read "退出程序"() -> (w244:bool)
        }
        n288 = call <vilib>:"DAQmx Clear Task.vi"("task in"=w61, "error in"=w64) -> ("error out"=w63:errorcluster)  [unwired: 13 in]
        n289 = call <vilib>:"Simple Error Handler.vi"("type of dialog (OK msg:1)"=w57, "error in (no error)"=w63) -> ()  [unwired: 3 in, 5 out]
        n290 = VISA Close(VISA resource name=w79, error in (no error)=w78) -> ()  [unwired: 1 out]
        n291 = node-c288(w52) -> ()  [unwired: 1 out]
        "电机已启动" <- FALSE
      }
    }
    n292 = local read "打开"() -> (w3:bool)
    n293 = And(x=w3, y="退出程序") -> (x .and. y?=w1:bool)
    n294 = case shown="False" w1 {
      frame False {
      }
      frame True {
        n295 = local write "打开"(FALSE ("打开")) -> ()
      }
    }
    "串口状态" <- "打开"
  }
